vi "write_headers_to_data_file.vi"(11 "file path in":path) -> (3 "file path out":path)   [LabVIEW 2016]
uses:
  <vilib>/Utility/file.llb/Write Delimited Spreadsheet (string).vi
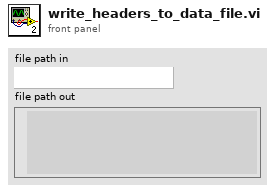
[diagram p1: front panel]
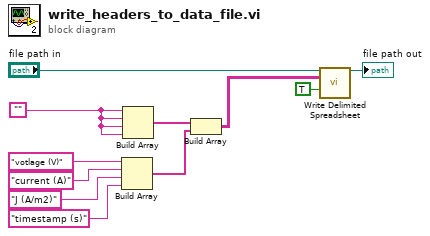
[diagram p0: block diagram]
diagram:
  w5 = ""
  n1 = Build Array("votlage (V)", "current (A)", "J (A/m2)", "timestamp (s)") -> (w3:string[])
  n2 = Build Array(w5, w5, w5, w5) -> (w4:string[])
  n3 = Build Array(w4, w3) -> (w2:string[][])
  n4 = call-poly <vilib>:"Write Delimited Spreadsheet.vi"("file path (dialog if empty)"="file path in", "2D data"=w2, "append to file? (new file:F)"=TRUE) -> ("new file path (Not A Path if cancelled)"=→"file path out":path)  [unwired: 11 in, 1 out]
